vi "IMU setup.vi"(8 "error in (no error)":errorcluster, 11 "Refnum in":T1) -> (0 "error out":errorcluster, 3 "Refnum out":T1)   [LabVIEW 2014]
uses:
  LabView/roger-i2c/Host API/Controls/FPGA I2C_FPGA Ref.ctl
  LabView/roger-i2c/Host API/I2C Host API.lvlib
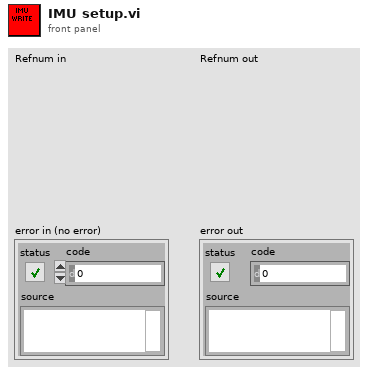
[diagram p1: front panel]
types:
  T1 = typedef "FPGA I2C_FPGA Ref.ctl" = refnum<k20>
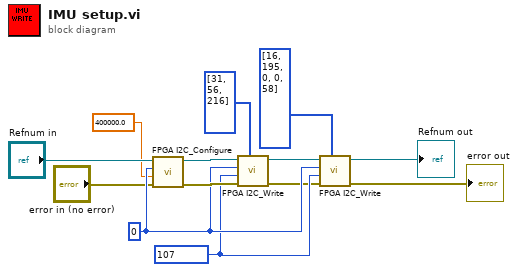
[diagram p0: block diagram]
diagram:
  w11 = u8 0 ("Port")
  w10 = u16 107 ("I2C_Address")
  n1 = call "FPGA I2C_Configure.vi"("error in"="error in (no error)", "Clock Rate (Hz)"=400000.0, "Port"=w11, "FPGA VI Reference"="Refnum in") -> ("error out"=w12:errorcluster, "FPGA VI Reference Out"=w13:T1)  [unwired: 6 out]
  n2 = call "FPGA I2C_Write.vi"("Write Data"=u8[] [31, 56, 216], "error in"=w12, "I2C_Address"=w10, "Port"=w11, "FPGA VI Reference"=w13) -> ("error out"=w6:errorcluster, "FPGA VI Reference Out"=w5:T1)  [unwired: 5 in]
  n3 = call "FPGA I2C_Write.vi"("Write Data"=u8[] [16, 195, 0, 0, 58], "error in"=w6, "I2C_Address"=w10, "Port"=w11, "FPGA VI Reference"=w5) -> ("error out"=→"error out":errorcluster, "FPGA VI Reference Out"=→"Refnum out":T1)  [unwired: 5 in]
